vi "delete_values.vi"(9 "F values array":dbl[][](array[numeric]), 10 "Frekans":dbl, 11 "LstBox Refnum":refnum<vi>) -> (3 "Output F values array":dbl[][](array[numeric]))   [LabVIEW 2014]
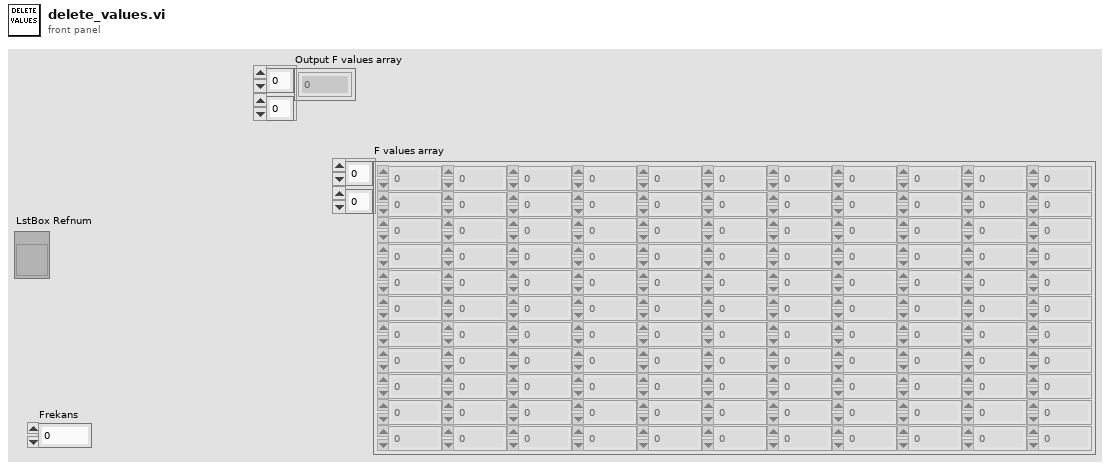
[diagram p1: front panel]
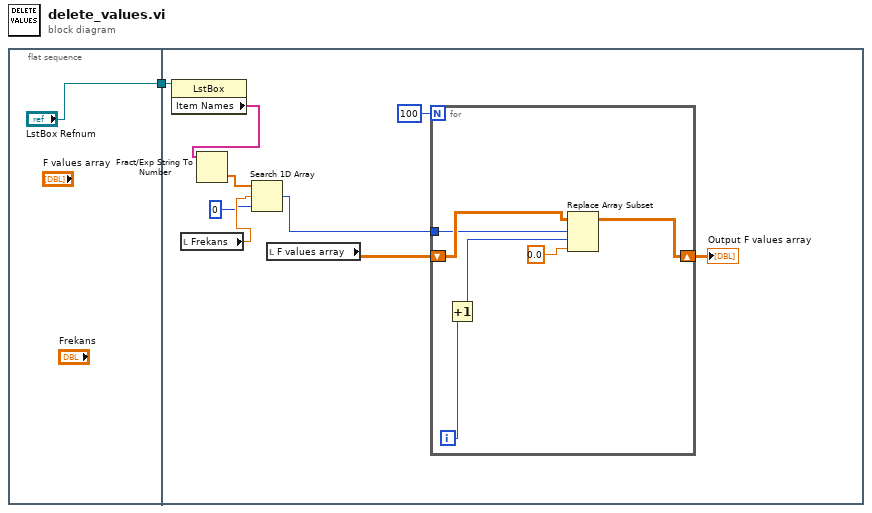
[diagram p0: block diagram]
diagram:
  n1 = flat-sequence {
    tunnel: ["LstBox Refnum"] -> w1
    tunnel: w1 -> [w5]
    frame #0 {
    }
    frame #1 {
      n2 = property class="LstBox"(reference=w5) -> ("Item Names"=w4:string[])  [unwired: 1 in, 2 out]
      n3 = local read "Frekans"() -> (w9:dbl)
      n4 = Fract/Exp String To Number(string=w4) -> (number=w10:dbl[])  [unwired: 3 in, 1 out]
      n5 = Search 1D Array(1D array=w10, element=w9, start index (0)=0) -> (index of element=w7:i32)
      n6 = local read "F values array"() -> (w11:dbl[][])
      n7 = for {
        N: 100 -> [_]
        shift-right: [w13] -> w3
        shift-left: w11 -> [w17]
        tunnel: w7 -> [w16]
        i -> [w14]
        n8 = Increment(x=w14) -> (x+1=w15:i32)
        n9 = Replace Array Subset(array=w17, new element=0.0 ("new element/subarray"), index (row)=w16, index (col)=w15) -> (w13:dbl[][])
      }
      "Output F values array" <- w3
    }
  }
